vi "Test.vi"() -> ()   [LabVIEW 2023]
uses:
  <vilib>/Utility/error.llb/DialogType.ctl
  <vilib>/ULx/Create Channel.llb/ULx Create Channel (DO-Digital Output).vi
  <vilib>/ULx/Write.llb/ULx Write (Digital 1D Bool 1Chan 1Samp).vi
panel:
  in  "lines":refnum<k21>
  in  "stop":bool
  in  "Data to write":bool[](array[boolean])
  in  "line grouping":i32(ring)=1 items=["OneChannelForEachLine", "OneChannelForAllLines"]
  # "Bits"
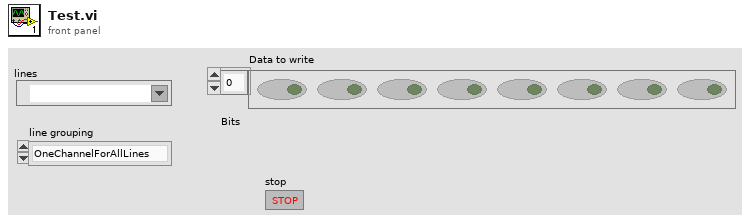
[diagram p1: front panel]
types:
  T1 = typedef "DialogType.ctl" = u16
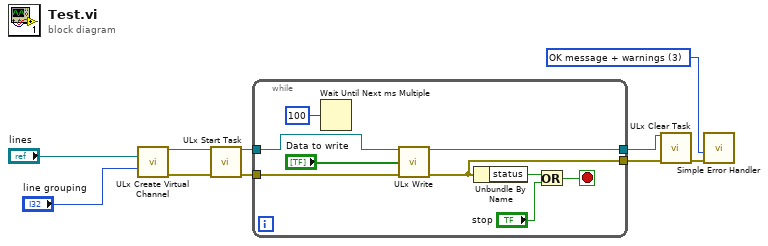
[diagram p0: block diagram]
diagram:
  w2 = T1 3 items=["no dialog", "OK message", "continue or stop message", "OK message + warnings", "continue/stop + warnings"] ("type of dialog (OK msg:1)")
  n1 = call-poly <vilib>:"ULx Create Virtual Channel.vi"("lines"="lines", "line grouping"="line grouping") -> ("task out"=w10:refnum<k24>, "error out"=w9:errorcluster)  [unwired: 12 in]
  n2 = call <vilib>:"ULx Start Task.vi"("task in"=w10, "error in"=w9) -> ("task out"=w7:refnum<k24>, "error out"=w6:errorcluster)  [unwired: 12 in]
  n3 = while {
    tunnel: w7 -> [w19]
    tunnel: w6 -> [w18]
    tunnel: [w16] -> w5
    tunnel: [w15] -> w4
    stop <- w14 stop-if-true
    n4 = Wait Until Next ms Multiple(millisecond multiple=u32 100 ("milliseconds to wait")) -> ()  [unwired: 1 out]
    n5 = call-poly <vilib>:"ULx Write.vi"("task in"=w19, "data"="Data to write", "error in"=w18) -> ("task out"=w16:refnum<k24>, "error out"=w15:errorcluster)  [unwired: 10 in, 1 out]
    n6 = Unbundle By Name(w15) -> ("status"=w12:bool)
    n7 = Or(x=w12, y="stop") -> (x .or. y?=w14:bool)
  }
  n8 = call <vilib>:"ULx Clear Task.vi"("task in"=w5, "error in"=w4) -> ("error out"=w3:errorcluster)  [unwired: 13 in]
  n9 = call <vilib>:"Simple Error Handler.vi"("type of dialog (OK msg:1)"=w2, "error in (no error)"=w3) -> ()  [unwired: 3 in, 5 out]
